vi "WhatDirection.vi"(1 "key":T1(ring)) -> (0 "direction":T1(ring))   [LabVIEW 2014]
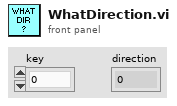
[diagram p1: front panel]
types:
  T1 = enum16{"0", "1", "2", "3", "4", "5", "6", "7", "8", "9", "A", "B", "C", "D", "E", "F", "G", "H", "I", "J", "K", "L", "M", "N", "O", "P", "Q", "R", "S", "T", "U", "V", "W", "X", "Y", "Z", "F1", "F2", "F3", "F4", "F5", "F6", "F7", "F8", "F9", "F10", "F11", "F12", "F13", "F14", "F15", "ADD", "BACK", "BACKSLASH", "CAPITAL", "COMMA", "DECIMAL", "DELETE", "DIVIDE", "DOWN", "END", "EQUALS", "ESCAPE", "GRAVE (`)", "HOME", "INSERT", "LBRACKET", "LCONTROL", "LEFT", "L ALT", "LSHIFT", "LWIN", "MINUS", "MULTIPLY", "NEXT", "NUMLOCK", "NUMPAD_0", "NUMPAD_1", "NUMPAD_2", "NUMPAD_3", "NUMPAD_4", "NUMPAD_5", "NUMPAD_6", "NUMPAD_7", "NUMPAD_8", "NUMPAD_9", "PAUSE", "PERIOD", "PRIOR (PG UP)", "RBRACKET", "RCONTROL", "RETURN", "RIGHT", "R ALT", "RSHIFT", "RWIN", "SCROLL", "SEMICOLON", "SLASH", "SPACE", "SUBTRACT", "TAB", "UP", "ENTER (num pad)", "' (quote)"}
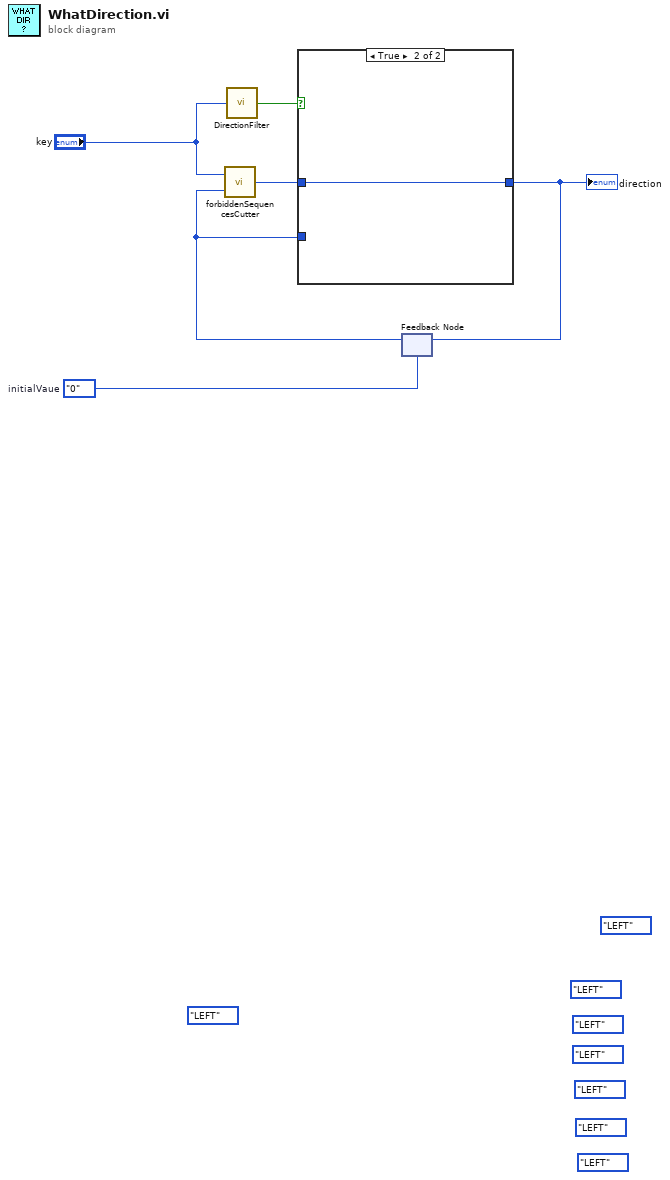
[diagram p0: block diagram]
diagram:
  (unwired) T1."LEFT" ("initialVaue")
  (unwired) T1."LEFT" ("initialVaue")
  (unwired) T1."LEFT" ("initialVaue")
  (unwired) T1."LEFT" ("initialVaue")
  (unwired) T1."LEFT" ("initialVaue")
  (unwired) T1."LEFT" ("initialVaue")
  (unwired) T1."LEFT" ("initialVaue")
  (unwired) T1."LEFT" ("initialVaue")
  w6 = T1."0"  # initialVaue
  n1 = call "DirectionFilter.vi"("keyType"="key") -> ("Result"=w4:bool)
  n2 = feedback #1(w6) -> (w1:T1)
  n3 = call "forbiddenSequencesCutter.vi"("initialVaue"=w1, "key  in"="key") -> ("key  out"=w3:T1)
  n4 = case shown="True" w4 {
    tunnel: w3 -> [_ w8]
    tunnel: [w7 w8] -> w5
    tunnel: w1 -> [w7 _]
    frame False {
    }
    frame True {
    }
  }
  "direction" <- w5
  n5 = feedback-in #1(w5) -> ()
